vi "Start.vi"(8 "error in (no error)":errorcluster, 10 "Message in":refnum<class "StartMessage.lvclass">=refnum, 11 "PockelCell in":refnum<class "PockelCell.lvclass">) -> (0 "error out":errorcluster, 3 "PockelCell out":refnum<class "PockelCell.lvclass">)   [LabVIEW 2012, in "PockelCell.lvclass"]
doc: "This member function is called when the statemachine in the run.vi receives an 'start' command. It relays the message to all observers of the component.\n\nOverride this member function in your derived class if you need additional start functionality (but don't forget to call the parent method)."
uses:
  PockelCell.lvclass
  <vilib>/Distrio/Murmex/GenericMessage/GenericMessage.lvclass
  Murmex/LabVIEW/Murmex/GenericMessage/GenericMessage.lvclass
  <vilib>/Distrio/Murmex/Murmex/Murmex.lvclass
  Murmex/LabVIEW/Murmex/StartMessage/StartMessage.lvclass
panel:
  # "This member function is called when the statemachine in the run.vi receives an 'start' command. It relays the message to all observers of the component.\n\nOverride this member function in your derived class if you need additional start functionality (but don't forget to call the parent method)."
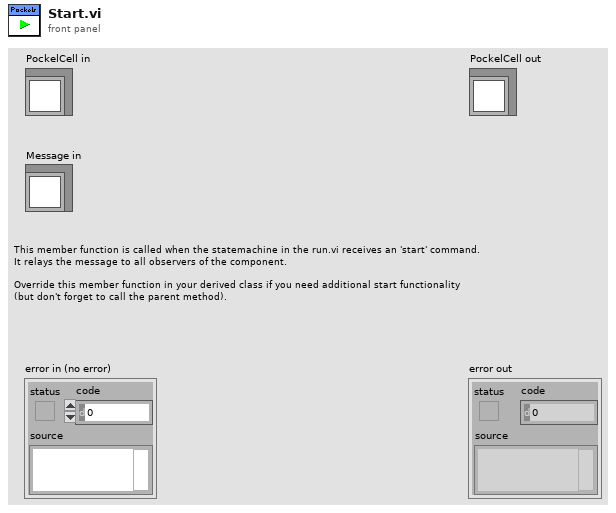
[diagram p1: front panel]
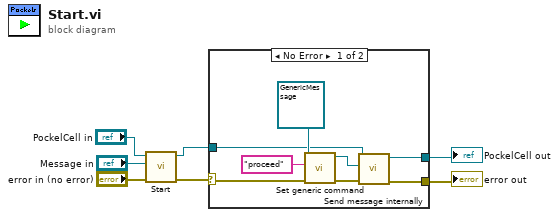
[diagram p0: block diagram]
diagram:
  n1 = call-parent "Start.vi"("error in (no error)"="error in (no error)", "Message in"="Message in", "Murmex in"="PockelCell in") -> ("error out"=w4:errorcluster, "Murmex out"=w2:refnum<class "PockelCell.lvclass">)  [unwired: 7 in]
  n2 = case shown="No Error" w4 {
    selector: w4 -> [w11 w16]
    tunnel: [w10 w16] -> w3
    tunnel: w2 -> [w9 w17]
    tunnel: [w8 w17] -> w1
    frame No Error {
      n3 = call <vilib>:"Set generic command.vi"("error in (no error)"=w11, "generic command"="proceed", "GenericMessage in"=refnum<class "GenericMessage.lvclass"> refnum ("GenericMessage.lvclass")) -> ("error out"=w14:errorcluster, "GenericMessage out"=w15:refnum<class "GenericMessage.lvclass">)  [unwired: 7 in]
      n4 = call "Send message internally.vi"("error in (no error)"=w14, "Message"=w15, "Murmex in"=w9) -> ("error out"=w10:errorcluster, "Murmex out"=w8:refnum<class "PockelCell.lvclass">)  [unwired: 7 in]
    }
    frame Error {
    }
  }
  "error out" <- w3
  "PockelCell out" <- w1
